vi "Get marker Name.vi"() -> (1 "Marker":string caption="Enter the Marker Text", 2 "Cancelled":bool)   [LabVIEW 2015]
uses:
  <vilib>/Utility/miscctls.llb/LVRectTypeDef.ctl
  <vilib>/Utility/inputDevices.llb/mouseAcquire.vi
panel:
  in  "Cancel":bool
  in  "OK":bool
  in  "Text":string caption="Enter the Marker Text"
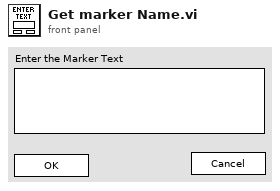
[diagram p1: front panel]
types:
  T1 = typedef "LVRectTypeDef.ctl" = cluster{"Left":i16, "Top":i16, "Right":i16, "Bottom":i16}
  T2 = cluster{"Horizontal":i32, "Vertical":i32, "Scrolling":i32}
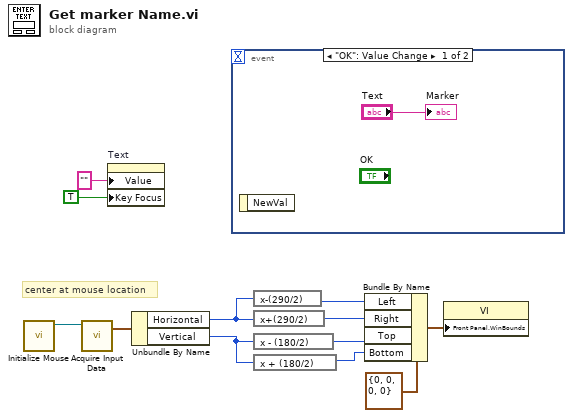
[diagram p0: block diagram]
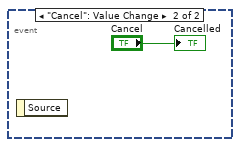
[diagram p2: hidden frame]
diagram:
  # "center at mouse location"
  n1 = call <vilib>:"Initialize Mouse.vi"() -> ("device ID"=w11:refnum<k1>)  [unwired: 10 in, 1 out]
  n2 = call-poly <vilib>:"Acquire Input Data.vi"("device ID"=w11) -> ("axis info"=w10:T2)  [unwired: 15 in, 3 out]
  n3 = property on="Text" class="Str"("Value"="" ("Text"), "Key Focus"=TRUE) -> ()  [unwired: 2 in, 2 out]
  n4 = Unbundle By Name(w10) -> ("Horizontal"=w3:i32, "Vertical"=w4:i32)
  n5 = event shown="[0] \"OK\": Value Change" {
    selector: _ -> [_ _]
    dyn-events: _ -> [_ _]
    timeout: _ -> [_ _]
    event "OK": Value Change {
      n6 = event-data() -> ()  [unwired: 1 in, 1 out]
      "Marker" <- "Text"
    }
    event "Cancel": Value Change {
      n7 = event-data() -> ()  [unwired: 1 in, 1 out]
      "Cancelled" <- "Cancel"
    }
  }
  n8 = expression code="x-(290/2)"(w3) -> (w7:i32)
  n9 = expression code="x+(290/2)"(w3) -> (w8:i32)
  n10 = expression code="x - (180/2)"(w4) -> (w6:i32)
  n11 = expression code="x + (180/2)"(w4) -> (w5:i32)
  n12 = Bundle By Name(cluster=T1 {"Left"=0, "Top"=0, "Right"=0, "Bottom"=0} ("Front Panel Window:Window Bounds"), "Left"=w7, "Right"=w8, "Top"=w6, "Bottom"=w5) -> (w2:T1)
  n13 = property class="VI"("Front Panel.WinBounds"=w2) -> ()  [unwired: 2 in, 2 out]
